vi "instantiate_qdrant_vector.vi"(0 "host_url":string, 5 "api_key":string, 11 "error in":errorcluster) -> (4 "vector_qdrant out":refnum<class "vector_qdrant.lvclass">, 15 "error out":errorcluster)   [LabVIEW 2020, in "vector_qdrant.lvclass"]
uses:
  vector_qdrant.lvclass
  vector_qdrant.lvclass/vector_qdrant.ctl
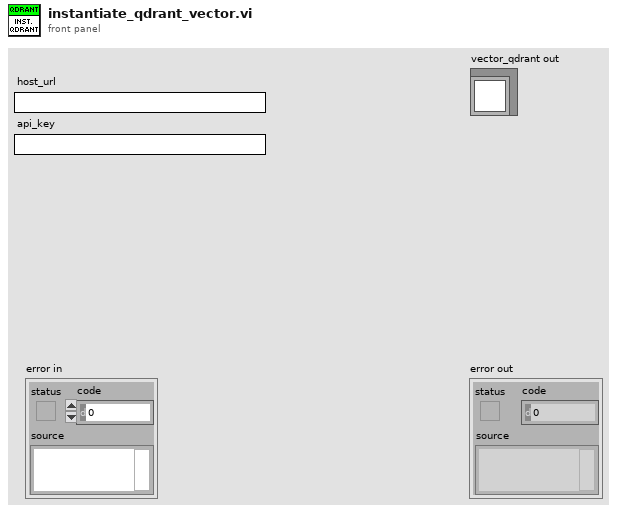
[diagram p1: front panel]
types:
  T1 = typedef "LabVIEWHTTPClient.lvlib/ClientHandle.ctl" = refnum<k1>
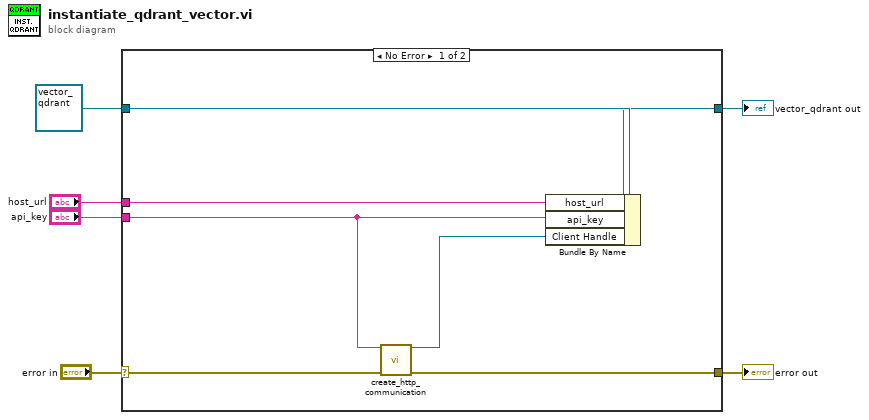
[diagram p0: block diagram]
diagram:
  n1 = case shown="No Error" "error in" {
    selector: "error in" -> [w10 w15]
    tunnel: [w9 w15] -> w5
    tunnel: [w12 w14] -> w3
    tunnel: refnum<class "vector_qdrant.lvclass"> refnum ("vector_qdrant in") -> [w13 w14]
    tunnel: "host_url" -> [w11 _]
    tunnel: "api_key" -> [w8 _]
    frame No Error {
      n2 = call "create_http_communication.vi"("api_key"=w8, "error in"=w10) -> ("client handle"=w7:T1, "error out"=w9:errorcluster)  [unwired: 12 in]
      n3 = Bundle By Name(cluster=w13, "host_url"=w11, "api_key"=w8, "Client Handle"=w7) -> (w12:refnum<class "vector_qdrant.lvclass">)
    }
    frame Error {
    }
  }
  "error out" <- w5
  "vector_qdrant out" <- w3
